vi "MonitoringOperationel.vi"() -> ()   [LabVIEW 2013]
panel:
  in  "Envoi":bool
  in  "data in":string
  out "?":bool
  in  "Afficher caractères reçus":bool
  in  "Log":bool
  out "error out":errorcluster
  out "Caractères reçus":string
  in  "Mode":T1(ring)=enum."CRLF"
  in  "?":bool
  in  "Tab Control":T2(tab)
  out "Signal Camera     ->    Fronts détectés":dbl[](graph)
  out "Signal Camera    ->  original":dbl[](graph)
  out "Moyenne":dbl
  out "?":dbl
  out "Position Servo":dbl(knob) scale=0.0..10.0
  out "Effective droite":dbl
  out "Consigne droite":dbl
  out "Effective gauche":dbl
  out "Consigne gauche":dbl
  out "Vitesse roue arrière droite [m/s]":dbl(knob) scale=0.0..10.0
  out "Vitesse roue arrière gauche [m/s]":dbl(knob) scale=0.0..10.0
  in  "PID 3.3":i8
  in  "PID 3.2":i8
  in  "PID Direction":i8
  in  "ABS":bool
  out "?":bool
  in  "PID vitesse":bool
  out "?":bool
  out "?":bool
  out "Array":bool[](array[boolean])
  in  "PID 2.3":i8
  in  "PID 2.2":i8
  in  "PID Léger":i8
  in  "PID 1.3":i8
  in  "PID 1.2":i8
  in  "PID Fort":i8
  # "Claudy essaie avec cette trame ça fonctionne parfaitement !"
  # "L:2F,34,34,35,35,35,37,38,3A,3B,3D,3F,40,42,44,46,48,49,4B,48,3C,45,6C,81,8D,8F,91,93,95,98,98,9B,9D,9F,9A,A0,A3,A7,A7,AA,AC,AD,B0,B2,B3,B5,B6,B8,B9,BA,BB,BC,BE,BE,C0,C1,C2,C2,C3,C3,C3,C4,C4,C4,C7,C7,C6,C4,C2,C2,C2,C1,C2,C1,C1,BF,BF,BD,BC,BB,B9,B8,B4,B2,AF,AD,A9,A8,A6,A6,A5,A5,A4,A2,A2,A0,9E,9B,9A,96,94,92,8F,8D,8B,89,87,84,82,80,7F,7D,7B,79,76,47,22,15,25,2F,33,32,32,30,2F,2E,2E,2D,2D,2C,2C,2B,2A,2A,28,27,25,24,22,22,1F,1E,11,85,85,80,81,80,80,82,81,82,81,82,82,81,82,82,82,82,81,82,7D,74,89,A7,95,8C,82,82,82,82,83,80,83,82,82,7B,86,83,84,80,83,82,81,83,82,81,82,81,82,81,81,81,81,82,80,82,81,81,80,81,80,80,81,80,80,83,80,7F,7E,7E,80,80,7F,81,7F,80,7E,80,7E,7F,7F,7E,7F,7C,7E,7D,7E,7C,7F,7E,80,7F,80,7F,7E,80,7E,7E,7D,7F,7C,7E,7E,7D,7E,7E,7E,7E,7D,7E,7E,7F,7E,7E,7E,7D,51,5B,73,90,8A,84,7F,80,7E,7F,7F,80,7F,80,7F,80,7F,7F,80,7E,7F,7E,7F,7E,80,7D,7F,7F,06,08,09,04,08,04,06,05,"
  # "Fort"
  # "Léger"
  # "Droite"
  # "Gauche"
  # "Fin"
  # "Perte Ligne"
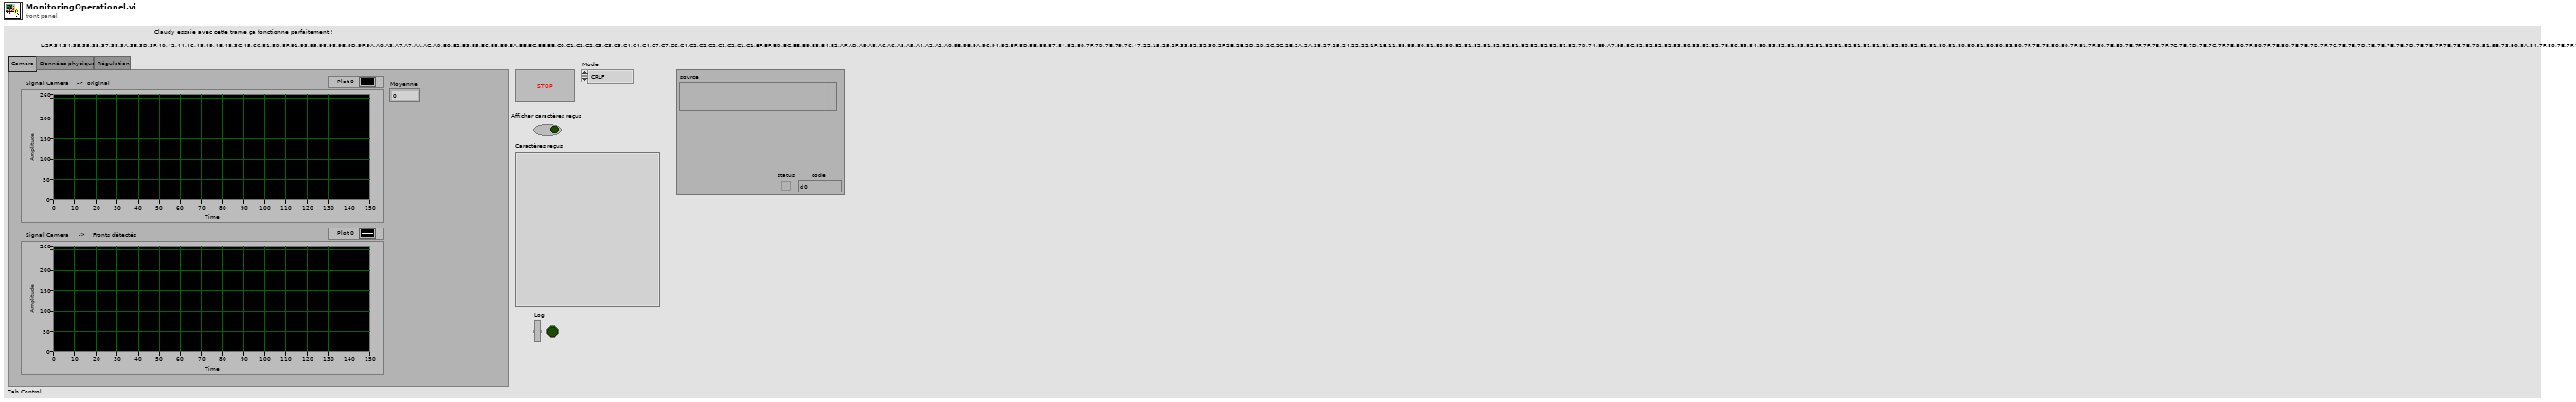
[diagram p1: front panel]
types:
  T1 = enum16{"Standard", "Buffered", "CRLF", "Immediate"}
  T2 = enum32{"Caméra", "Données physique", "Régulation"}
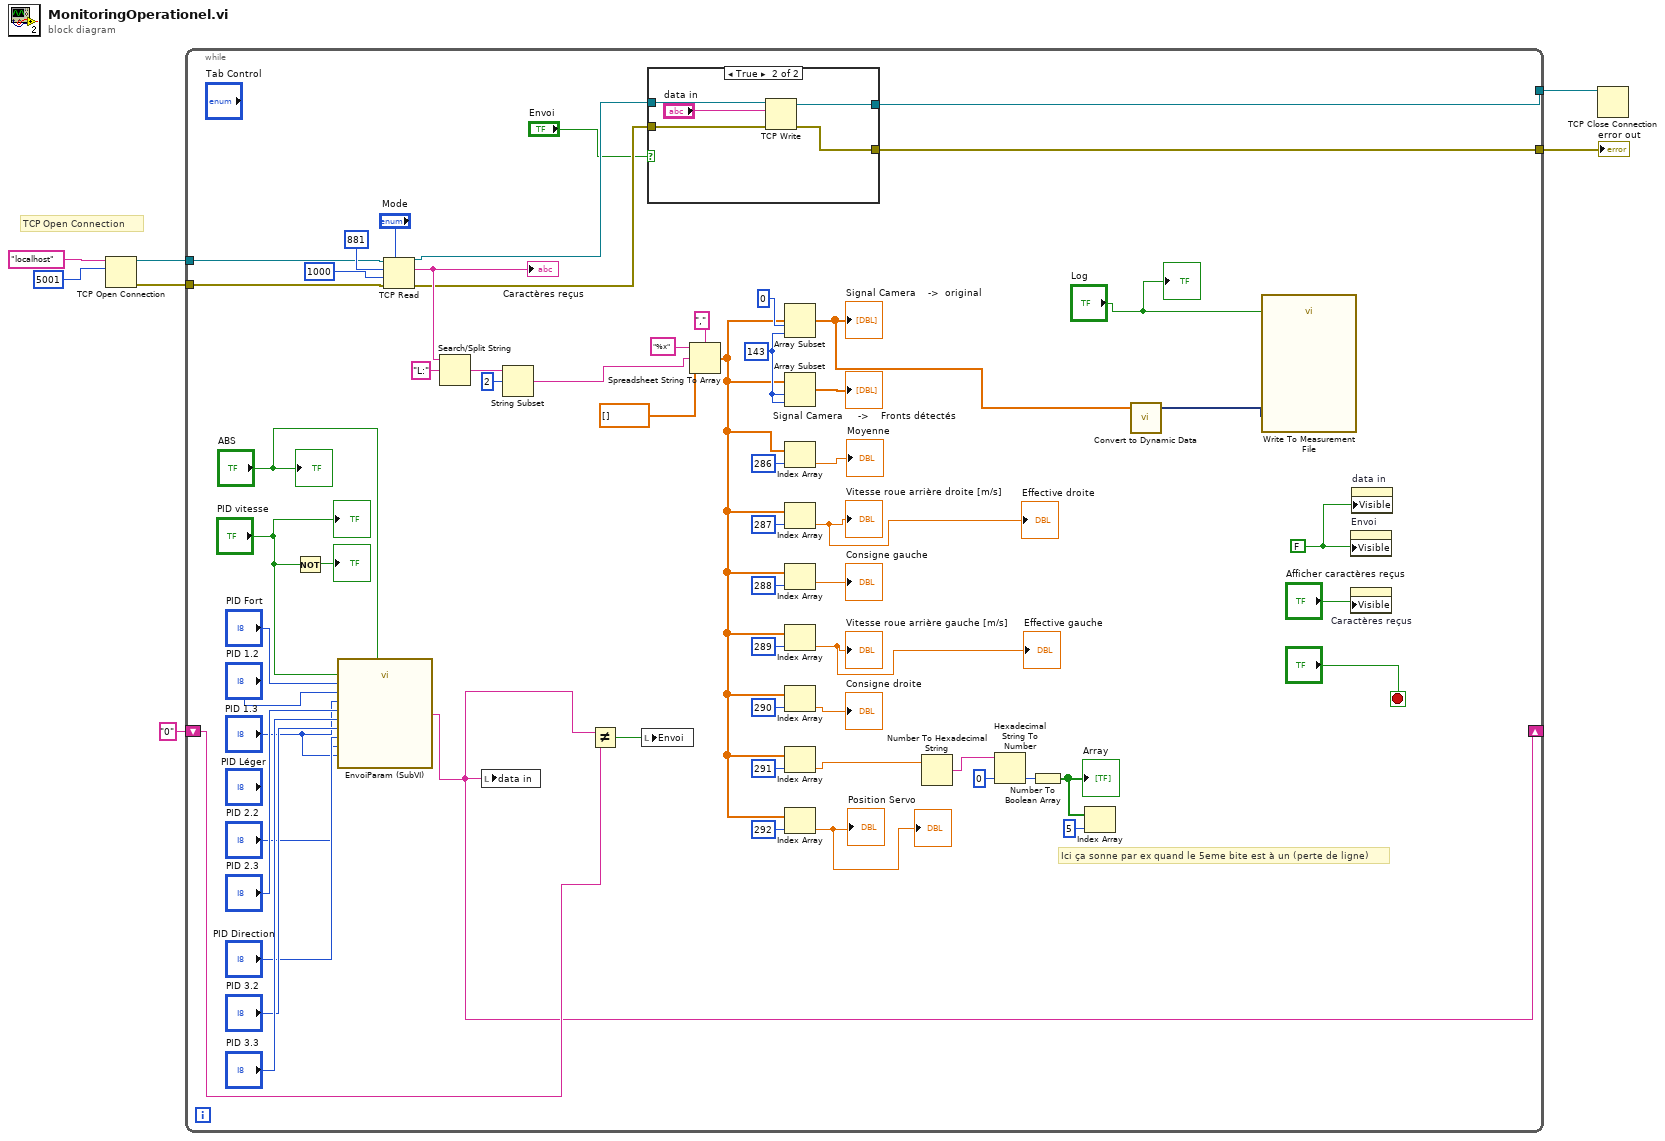
[diagram p0: block diagram]
diagram:
  # "TCP Open Connection"
  n1 = TCP Open Connection(address="localhost", remote port or service name=u16 5001) -> (connection ID=w5:refnum<k5>, error out=w4:errorcluster)  [unwired: 3 in]
  n2 = while {
    tunnel: w5 -> [w42]
    tunnel: w4 -> [w55]
    tunnel: [w40] -> w3
    tunnel: [w38] -> w2
    shift-right: [w24] -> _
    shift-left: "0" -> [w35]
    stop <- "?" stop-if-true
    w36 = FALSE
    w54 = 143 ("length")
    # "Ici ça sonne par ex quand le 5eme bite est à un (perte de ligne)"
    n3 = Not(x="PID vitesse") -> (.not. x?=→"?":bool)
    n4 = call "EnvoiParam (SubVI).vi"("PID 3.3"="PID 3.3", "PID 3.2"="PID 3.2", "PID Direction"="PID Direction", "PID 2.3"="PID 2.3", "PID 2.2"="PID 2.2", "PID Léger"="PID 1.3", "PID 1.3"="PID 1.3", "PID 1.2"="PID 1.2", "PID Fort"="PID Fort", "PID vitesse"="PID vitesse", "ABS"="ABS") -> ("String"=w24:string)
    n5 = TCP Read(connection ID=w42, bytes to read=881, error in (no error)=w55, 7:"Mode", 9:1000 ("timeout ms (25000)")) -> (connection ID out=w41:refnum<k5>, data out=w63:string, error out=w39:errorcluster)
    "Caractères reçus" <- w63
    n6 = Search/Split String(string=w63, search string/char (-)="L:") -> (match + rest of string=w61:string)  [unwired: 1 in, 2 out]
    n7 = local write "data in"(w24) -> ()
    n8 = String Subset(string=w61, offset (0)=2) -> (substring=w62:string)  [unwired: 1 in]
    n9 = Not Equal?(x=w24, y=w35) -> (x != y?=w34:bool)
    n10 = local write "Envoi"(w34) -> ()
    n11 = case shown="True" "Envoi" {
      tunnel: w41 -> [w70 w75]
      tunnel: [w70 w74] -> w40
      tunnel: w39 -> [w69 w73]
      tunnel: [w69 w72] -> w38
      frame False {
      }
      frame True {
        n12 = TCP Write(connection ID=w75, data in="data in", error in (no error)=w73) -> (connection ID out=w74:refnum<k5>, error out=w72:errorcluster)  [unwired: 1 in, 1 out]
      }
    }
    n13 = Spreadsheet String To Array(delimiter (Tab)=",", format string="%x", spreadsheet string=w62, array type (2D Dbl)=dbl[] []) -> (array=w13:dbl[])
    n14 = Array Subset(array=w13, index=0, length=w54) -> (w47:dbl[])
    "Signal Camera    ->  original" <- w47
    n15 = Array Subset(array=w13, index=w54, length=w54) -> (→"Signal Camera     ->    Fronts détectés":dbl[])
    n16 = Index Array(array=w13, index=286) -> (element=→"Moyenne":dbl)
    n17 = Index Array(array=w13, index=287) -> (element=→"Effective droite" →"Vitesse roue arrière droite [m/s]":dbl)
    n18 = Index Array(array=w13, index=288) -> (element=→"Consigne gauche":dbl)
    n19 = Index Array(array=w13, index=289) -> (element=→"Vitesse roue arrière gauche [m/s]" →"Effective gauche":dbl)
    n20 = Index Array(array=w13, index=290) -> (element=→"Consigne droite":dbl)
    n21 = Index Array(array=w13, index=291) -> (element=w17:dbl)
    n22 = Index Array(array=w13, index=292) -> (element=→"Position Servo" →"?":dbl)
    n23 = Number To Hexadecimal String(2:w17) -> (0:w50:string)  [unwired: 1 in]
    n24 = Hexadecimal String To Number(string=w50, default (0uL)=u8 0 ("default (0 U32)")) -> (number=w51:u8)  [unwired: 1 in, 1 out]
    n25 = Number To Boolean Array(number=w51) -> (Boolean array=w49:bool[])
    "Array" <- w49
    n26 = Index Array(array=w49, index=5) -> ()  [unwired: 1 out]
    n27 = call "Convert to Dynamic Data"("Array"=w47) -> ("Dynamic Data Type"=w45:dynamicdata)  [unwired: 3 in]
    n28 = call "Write To Measurement File"("Signals"=w45, "Enable"="Log") -> ()  [unwired: 15 in, 3 out]
    n29 = property on="Envoi" class="Bool (strict)"("Visible"=w36) -> ()  [unwired: 2 in, 2 out]
    n30 = property on="Caractères reçus" class="Str"("Visible"="Afficher caractères reçus") -> ()  [unwired: 2 in, 2 out]
    n31 = property on="data in" class="Str"("Visible"=w36) -> ()  [unwired: 2 in, 2 out]
    "?" <- "ABS"
    "?" <- "PID vitesse"
    "?" <- "Log"
  }
  "error out" <- w2
  n32 = TCP Close Connection(connection ID=w3) -> ()  [unwired: 2 in, 2 out]
